vi "Test Channel Array Size Error.vi"(8 "error in (no error)":errorcluster, 11 "Scan Engine Scripting API Modules in":refnum<class "Scan Engine Scripting API Modules.lvclass">) -> (0 "error out":errorcluster, 3 "Scan Engine Scripting API Modules out":refnum<class "Scan Engine Scripting API Modules.lvclass">)   [LabVIEW 2020, in "Scan Engine Scripting API Modules.lvclass"]
uses:
  Scan Engine Scripting API Modules.lvclass
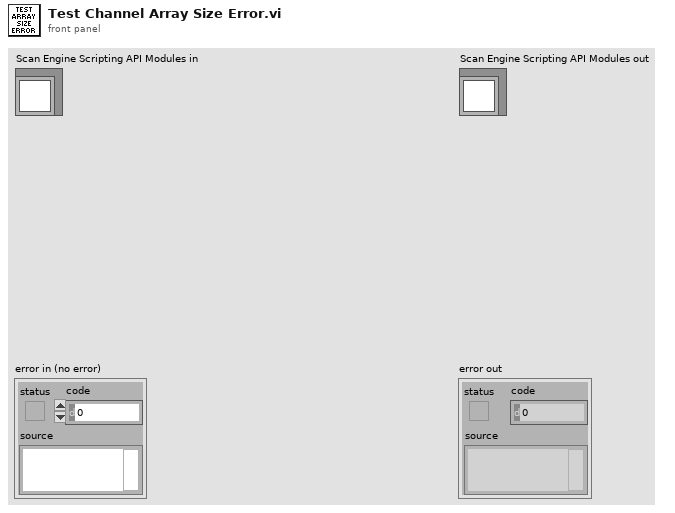
[diagram p1: front panel]
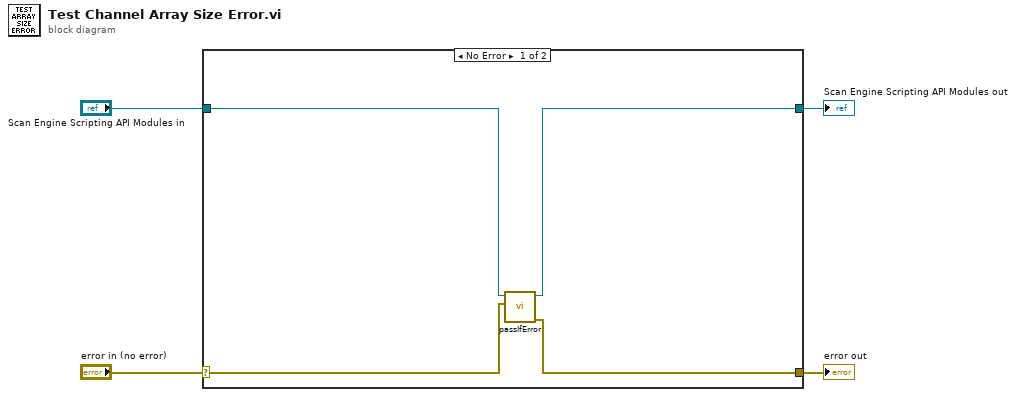
[diagram p0: block diagram]
diagram:
  n1 = case shown="No Error" "error in (no error)" {
    selector: "error in (no error)" -> [w5 w10]
    tunnel: [w8 w10] -> w3
    tunnel: [w6 w9] -> w1
    tunnel: "Scan Engine Scripting API Modules in" -> [w7 w9]
    frame No Error {
      n2 = call-dynamic "passIfError.vi"("error"=w5, "TestCase in"=w7) -> ("error out"=w8:errorcluster, "TestCase out"=w6:refnum<class "Scan Engine Scripting API Modules.lvclass">)  [unwired: 8 in]
    }
    frame Error {
    }
  }
  "error out" <- w3
  "Scan Engine Scripting API Modules out" <- w1
